vi "GenerateT1Mask.vi"(6 "Mask Selector":u16(ring)=1 items=["ITU", "EIA/TIA 547-1989"], 8 "error in (no error)":errorcluster, 9 "Reset":bool, 10 "Polarity":bool, 11 "Waveform":waveform(dbl)) -> (0 "error out":errorcluster, 2 "test passed?":bool, 3 "output values":waveform(dbl)[](array[waveform]))   [LabVIEW 2018]
doc: "Generate T1 Mask"
uses:
  <vilib>/measure/mamon.llb/Create Continuous Mask.vi
  <vilib>/measure/mamon.llb/Trigger Detection for 1 Channel.vi
  Align Mask and Signal - cluster.vi
  <vilib>/measure/mamon.llb/Limit Testing Time.vi
  <vilib>/measure/NI_MAPro.lvlib
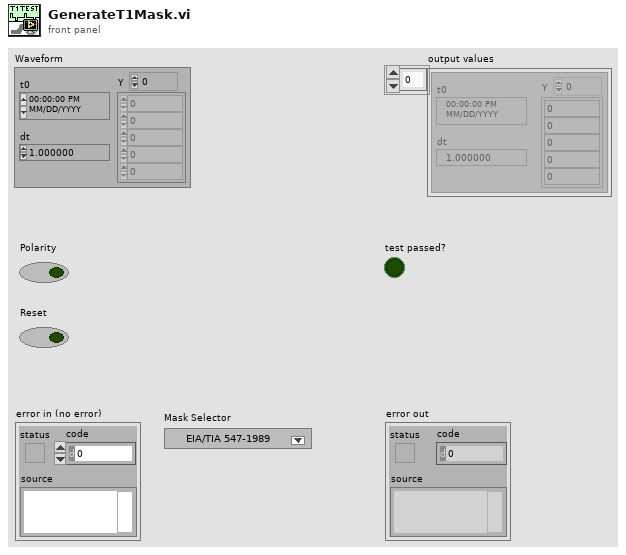
[diagram p1: front panel]
types:
  T1 = cluster{"ANSI X High":dbl[], "ANSI Y High":dbl[]}
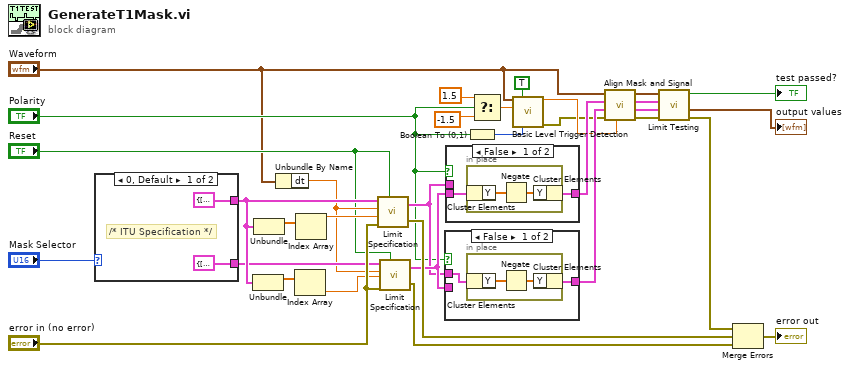
[diagram p0: block diagram]
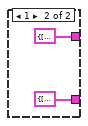
[diagram p4: hidden frame]
diagram:
  n1 = case shown="0, Default" "Mask Selector" {
    tunnel: [cluster{"ITU X High":dbl[], "ITU Y High":dbl[]} {"ITU X High"=[-3.238341e-07, -2.428756e-07, -1.86917e-07, -1.85917e-07, 1.85917e-07, 1.86917e-07, 2.428756e-07, 3.23834e-07], "ITU Y High"=[0.15, 0.15, 1.5, 3.7, 3.7, 1.5, 0.15, 0.15]} ("ITU Upper Specification Cluster") T1 {"ANSI X High"=[-3.238341e-07, -2.5e-07, -1.75e-07, -1.74e-07, -7.5e-08, 0.0, 1.75e-07, 2.25e-07, 3.75e-07], "ANSI Y High"=[0.05, 0.05, 0.8, 1.15, 1.15, 1.05, 1.05, -0.07, 0.05]} ("EIA/TIA Upper Specification Cluster")] -> w26
    tunnel: [cluster{"ITU X Low":dbl[], "ITU Y Low":dbl[]} {"ITU X Low"=[-3.238341e-07, -1.36917e-07, -1.35917e-07, 0.0, 8.09585e-08, 1.35917e-07, 1.36917e-07, 2.158894e-07, 3.238341e-07], "ITU Y Low"=[-0.15, -0.15, 1.5, 2.3, 2.3, 1.5, -1.2, -1.2, -0.15]} ("ITU Lower Specification Cluster") cluster{"ANSI X Low":dbl[], "ANSI Y Low":dbl[]} {"ANSI X Low"=[-3.238341e-07, -1.5e-07, -1.49e-07, -1e-07, 0.0, 1e-07, 1.49e-07, 1.5e-07, 3e-07, 4.25e-07], "ANSI Y Low"=[-0.05, -0.05, 0.5, 0.95, 0.95, 0.9, 0.5, -0.45, -0.45, -0.2]} ("EIA/TIA Lower Specification Cluster")] -> w25
    frame 0, Default {
      # "/* ITU Specification */"
    }
    frame 1 {
    }
  }
  n2 = Unbundle(w26) -> ("ANSI X High"=w28:dbl[])  [unwired: 1 out]
  n3 = Unbundle(w26) -> ("ANSI X High"=w30:dbl[])  [unwired: 1 out]
  n4 = Unbundle By Name("Waveform") -> ("dt"=w22:dbl)
  n5 = Index Array(array=w28) -> (element=w27:dbl)  [unwired: 1 in]
  n6 = Index Array(array=w30) -> (element=w29:dbl)  [unwired: 1 in]
  n7 = call-poly <vilib>:"Limit Specification.vi"("Specification Cluster"=w26, "dx"=w22, "x0"=w29, "error in (no error)"="error in (no error)", "Reset"="Reset") -> ("Limit"=w19:cluster{"x0":dbl, "dx":dbl, "Y":dbl[]}, "error out"=w24:errorcluster)
  n8 = call-poly <vilib>:"Limit Specification.vi"("Specification Cluster"=w25, "dx"=w22, "x0"=w27, "error in (no error)"="error in (no error)", "Reset"="Reset") -> ("Limit"=w20:cluster{"x0":dbl, "dx":dbl, "Y":dbl[]}, "error out"=w23:errorcluster)
  n9 = case shown="False" "Polarity" {
    tunnel: w20 -> [_ w42]
    tunnel: [w39 w42] -> w14
    tunnel: w19 -> [w38 _]
    frame False {
      n10 = in-place {
        n11 = in-place-cluster #1(w38) -> ("Y"=w41:dbl[])
        n12 = Negate(x=w41) -> (-x=w40:dbl[])
        n13 = in-place-cluster #1("Y"=w40) -> (w39:cluster{"x0":dbl, "dx":dbl, "Y":dbl[]})
      }
    }
    frame True {
    }
  }
  n14 = case shown="False" "Polarity" {
    tunnel: [w43 w47] -> w15
    tunnel: w19 -> [_ w47]
    tunnel: w20 -> [w44 _]
    frame False {
      n15 = in-place {
        n16 = in-place-cluster #2(w44) -> ("Y"=w46:dbl[])
        n17 = Negate(x=w46) -> (-x=w45:dbl[])
        n18 = in-place-cluster #2("Y"=w45) -> (w43:cluster{"x0":dbl, "dx":dbl, "Y":dbl[]})
      }
    }
    frame True {
    }
  }
  n19 = Boolean To (0,1)(Boolean="Polarity") -> (0, 1=w5:i16)
  n20 = Select(t=1.5, s="Polarity", f=-1.5) -> (s? t:f=w8:dbl)
  n21 = call-poly <vilib>:"Basic Level Trigger Detection.vi"("signal in"="Waveform", "reset"=TRUE ("Reset"), "level"=w8, "trigger slope"=w5) -> ("trigger location"=w4:dbl, "error out"=w3:errorcluster)  [unwired: 9 in, 1 out]
  n22 = call-poly "Align Mask and Signal.vi"("trigger index"=w4, "error in (no error)"=w3, "lower limit"=w14, "upper limit"=w15, "Waveform"="Waveform") -> ("error out"=w2:errorcluster, "lower limit out"=w11:cluster{"x0":dbl, "dx":dbl, "Y":dbl[]}, "upper limit out"=w12:cluster{"x0":dbl, "dx":dbl, "Y":dbl[]}, "Waveform out"=w13:waveform(dbl))  [unwired: 2 in, 1 out]
  n23 = call-poly <vilib>:"Limit Testing.vi"("error in (no error)"=w2, "lower limit"=w11, "upper limit"=w12, "signal in"=w13) -> ("error out"=w1:errorcluster, "output values"=→"output values":waveform(dbl)[], "test passed?"=→"test passed?":bool)  [unwired: 2 in, 3 out]
  n24 = Merge Errors(w1, w24, w23) -> (→"error out":errorcluster)
